vi "Open Reentrant Class Method VI.vi"(8 "error in (no error)":errorcluster, 10 "Method VI Filename to Open":path, 11 "Generic Plugin in":refnum<class "Generic Plugin.lvclass">) -> (0 "error out":errorcluster, 3 "VI Refnum":refnum<vi>)   [LabVIEW 2020, in "RxnRover.lvlib" / "Generic Plugin.lvclass"]
doc: "Opens a class method VI reference for reentrant execution. This VI is intented to work both in the development environment and in stand-alone programs."
uses:
  Generic Plugin.lvclass
  File IO/File IO.lvlib
  logging/logging.lvlib
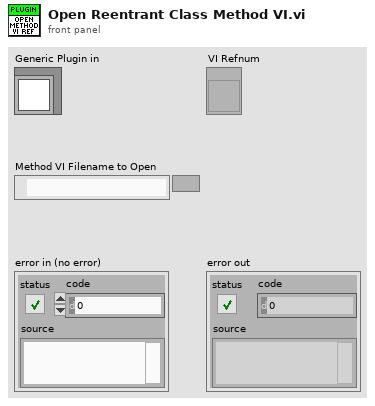
[diagram p1: front panel]
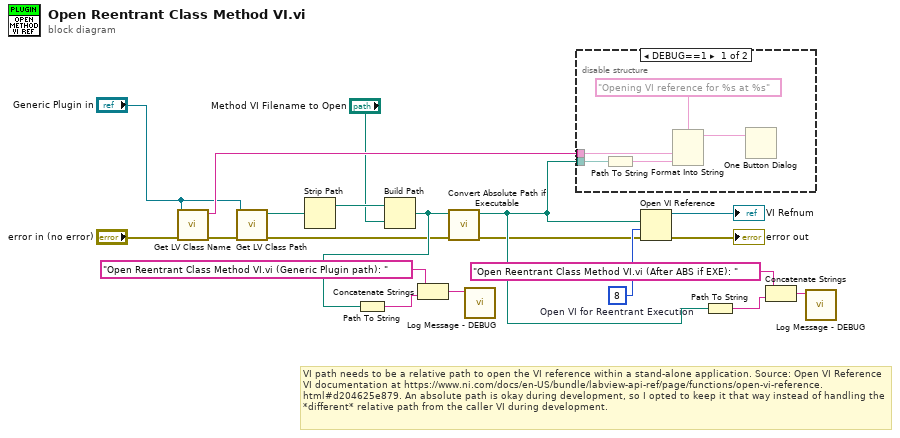
[diagram p0: block diagram]
diagram:
  w14 = 8  # Open VI for Reentrant Execution
  # "VI path needs to be a relative path to open the VI reference within a stand-alone application. Source: Open VI Reference VI documentation at https://www.ni.com/docs/en-US/bundle/labview-api-ref/page/functions/open-vi-reference.html#d204625e879. An absolute path is okay during development, so I opted to keep it that way instead of handling the *different* relative path from the caller VI during development."
  n1 = call <vilib>:"Get LV Class Name.vi"("error in (no error)"="error in (no error)", "object"="Generic Plugin in") -> ("error out"=w19:errorcluster, "class name"=w20:string)  [unwired: 8 in]
  n2 = call <vilib>:"Get LV Class Path.vi"("error in (no error)"=w19, "object"="Generic Plugin in") -> ("error out"=w1:errorcluster, "class path"=w8:path)  [unwired: 8 in]
  n3 = Strip Path(path=w8) -> (stripped path=w16:path)  [unwired: 1 out]
  n4 = Build Path(base path=w16, name or relative path="Method VI Filename to Open") -> (appended path=w4:path)
  n5 = Path To String(path=w4) -> (string=w9:string)
  n6 = Concatenate Strings("Open Reentrant Class Method VI.vi (Generic Plugin path): " ("string"), w9) -> (w11:string)
  n7 = call "Convert Absolute Path if Executable.vi"("error in (no error)"=w1, "Absolute Path"=w4) -> ("error out"=w2:errorcluster, "Result Path"=w3:path)  [unwired: 7 in, 1 out]
  n8 = call "Log Message - DEBUG.vi"("Message"=w11) -> ()  [unwired: 10 in, 1 out]
  n9 = disable-structure shown="DEBUG==1" {
    disable-tunnel: w3 -> [w25 _]
    disable-tunnel: w20 -> [w21 _]
    frame condition #0 {
      n10 = Path To String(path=w25) -> (string=w22:string)
      n11 = Format Into String(format string="Opening VI reference for %s at %s", w21, w22) -> (resulting string=w23:string)  [unwired: 2 in, 1 out]
      n12 = One Button Dialog(message=w23) -> ()  [unwired: 1 in, 1 out]
    }
    frame condition #1 (active) {
      # "Do nothing"
    }
  }
  n13 = Open VI Reference(vi path=w3, options=w14, error in (no error)=w2) -> (vi reference=→"VI Refnum":refnum<vi>, error out=→"error out":errorcluster)  [unwired: 3 in]
  n14 = Path To String(path=w3) -> (string=w5:string)
  n15 = Concatenate Strings("Open Reentrant Class Method VI.vi (After ABS if EXE): " ("string"), w5) -> (w7:string)
  n16 = call "Log Message - DEBUG.vi"("Message"=w7) -> ()  [unwired: 10 in, 1 out]
